vi "Get_Sweep_Status.vi"(8 "error in (no error)":errorcluster, 11 ".NET Reference in":refnum<k24>) -> (0 "error out":errorcluster, 2 "status":i32(ring) items=["Standby", "Running", "Pausing", "WaitingforTrigger", "Returning", ""], 3 "Reference out":refnum<k24>)   [LabVIEW 2017]
uses:
  D:/test/FULLband-sts/Fullband_Sample/DLL/InstrumentDLL.dll
  DLL/InstrumentDLL.dll
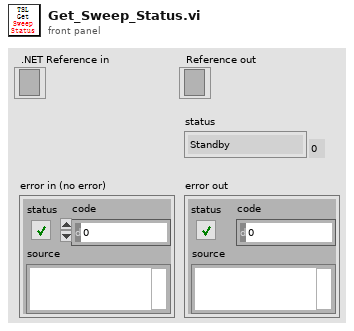
[diagram p1: front panel]
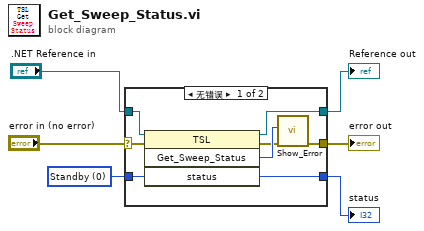
[diagram p0: block diagram]
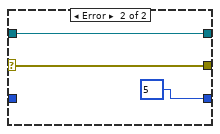
[diagram p2: hidden frame]
diagram:
  w2 = 0 items=["Standby", "Running", "Pausing", "WaitingforTrigger", "Returning"] ("status")
  n1 = case shown="无错误" "error in (no error)" {
    selector: "error in (no error)" -> [w7 w17]
    tunnel: [w14 w15] -> w6
    tunnel: ".NET Reference in" -> [w13 w16]
    tunnel: [w12 w16] -> w4
    tunnel: [w8 w17] -> w3
    tunnel: w2 -> [w11 _]
    frame No Error {
      n2 = invoke on="调用节点" class="TSL" method="Get_Sweep_Status"(reference=w13, error in=w7, "status"=w11) -> (reference out=w12:refnum<k24>, error out=w9:errorcluster, "Get_Sweep_Status"=w10:i32, "status"=w14:i32)  [unwired: 1 in]
      n3 = call "Show_Error.vi"("error in (no error)"=w9, "Error"=w10) -> ("error out"=w8:errorcluster)  [unwired: 9 in]
    }
    frame Error {
      w15 = 5 items=["Standby", "Running", "Pausing", "WaitingforTrigger", "Returning", ""] ("status")
    }
  }
  "Reference out" <- w4
  "error out" <- w3
  "status" <- w6
